vi "Read PWM Output Channel.vi"(8 "error in":errorcluster, 11 "PWM output channel in":refnum<class "PWM Output Channel.lvclass">) -> (0 "error out":errorcluster, 1 "default value":dbl, 2 "name":string, 3 "PWM output channel out":refnum<class "PWM Output Channel.lvclass">, 4 "index":i32, 5 "frequency":T1)   [LabVIEW 2020, in "Scan Engine Scripting.lvlib" / "PWM Output Channel.lvclass"]
uses:
  PWM Output Channel.lvclass
  Frequency.ctl
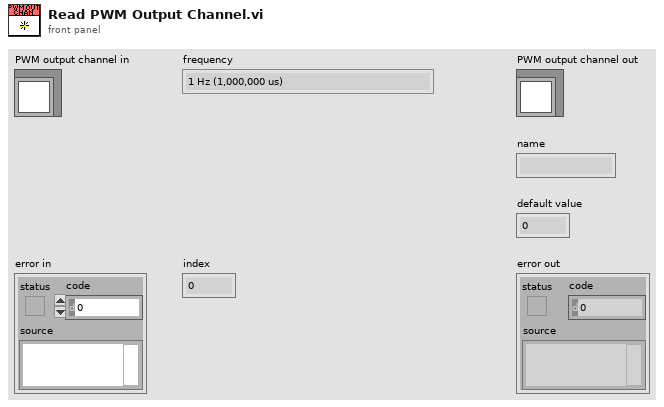
[diagram p1: front panel]
types:
  T1 = typedef "Scan Engine Scripting.lvlib/PWM Output Channel.lvclass/Frequency.ctl" = enum16{"1 Hz (1,000,000 us)", "50 Hz (20,000 us)", "250 Hz (4,000 us)", "500 Hz (2,000 us)", "1 kHz (1,000 us)", "5 kHz (200 us)", "10 kHz (100 us)", "20 kHz (50 us)"}
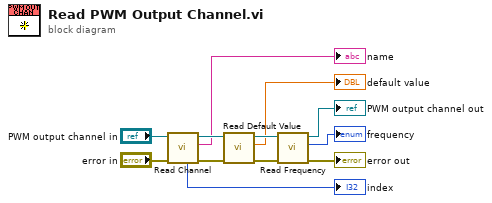
[diagram p0: block diagram]
diagram:
  n1 = call-dynamic "Read Channel.vi"("error in"="error in", "channel in"="PWM output channel in") -> ("error out"=w10:errorcluster, "name"=→"name":string, "channel out"=w9:refnum<class "PWM Output Channel.lvclass">, "index"=→"index":i32)  [unwired: 4 in, 2 out]
  n2 = call-dynamic "Read Default Value.vi"("error in"=w10, "PWM channel in"=w9) -> ("error out"=w8:errorcluster, "default value"=→"default value":dbl, "PWM channel out"=w7:refnum<class "PWM Output Channel.lvclass">)  [unwired: 7 in]
  n3 = call-dynamic "Read Frequency.vi"("error in"=w8, "PWM output channel in"=w7) -> ("error out"=→"error out":errorcluster, "frequency"=→"frequency":T1, "PWM output channel out"=→"PWM output channel out":refnum<class "PWM Output Channel.lvclass">)  [unwired: 7 in]
